vi "AlliGator n-Exp + IRF Fit v4.vi"(0 "Decay":cluster{"t Array":dbl[], "Data Array":dbl[]}, 1 "VI Refnum":refnum<vi>, 5 "IRF":cluster{"t Array":dbl[], "IRF Array":dbl[]}, 7 "Fit Options":T13={"Show Fit Residuals"=TRUE, "Fit Model"=enum."1-Exponential", "Residual Type"=enum."Standard", "Max Decay Percentile"=0.0, "Min Decay Percentile"=0.0, "Show Full Decay"=TRUE, "Weights"=enum."Unweighted", "Fitting Method"=enum."Least Square", "Compute Parameter Uncertainties"=TRUE, "Periodic Boundaries"=TRUE, "Model Calculation"=enum."Simulation", "Period"=1.2500000000000001e-08, "Termination Criteria"={"Max Iterations"=1000, "Max Function Calls"=0, "Max Time"=1000.0, "Function Tolerance"=1e-06, "Parameter Tolerance"=1e-06, "Gradient Tolerance"=0.0, "Min Lambda"=1e-06, "Max Lambda"=1e-06, "Initial Tick Count"=0}, "Offset Resolution"=1.2500000000000001e-08, "Use Local IRF"=TRUE, "Fitting Algorithm"=enum."Levenberg-Marquardt"} {"Offset Resolution" min=0.0; "Period" min=0.0; "Min Decay Percentile" min=0.0 max=1.0; "Max Decay Percentile" min=0.0 max=1.0}, 9 "MLE Fit Options":T1, 11 "error in (no error)":errorcluster, 12 "All Parameter Constraints":T10) -> (3 "All unscaled Fit Parameters (w tau)":dbl[](array[numeric]), 4 "Fitted Decay":cluster{"t Array":dbl[], "Fitted Array":dbl[]}, 6 "Residuals":cluster{"t Array":dbl[], "Residual Array":dbl[]}, 8 "Fit Output":T4={"best nonlinear fit"=[], "best fit parameters"=[], "R^2"=0.0, "RMSE"=0.0, "error out"={"status"=FALSE, "code"=0, "source"=""}, "Fitting Method"=enum."Least Square", "number of function calls"=0, "number of iterations"=0, "covariance"=[], "Chi 2"=0.0, "DOF"=0, "Fit Convergence Criterion"=enum."Continue", "Fitting Algorithm"=enum."Levenberg-Marquardt", "Weighted Fit"=FALSE, "Gradient"=0.0, "|Delta Chi 2|"=0.0, "|Delta Chi 2|/Chi 2"=0.0, "Max |Delta a| /|a|"=0.0, "Lambda"=-1.0, "RSS"=0.0, "AIC"=0.0, "BIC"=0.0, "Max number of function calls"=0, "Max number of iterations"=0, "IRF"={"X Array"=[], "Y Array"=[]}, "IRF Normalization Factor"=0.0, "Decay Normalization Factor"=0.0}, 10 "Delta Best Fit Parameters (w tau)":dbl[](array[numeric]), 13 "Guess Parameters Options":T3=enum."User-provided (normalized)", 14 "Guess Parameters":dbl[](array[numeric]), 15 "error out":errorcluster)   [LabVIEW 2021, in "AlliGator Decay Analysis.lvlib" / "AlliGator Decay Fit.lvlib"]
doc: "Fits the provided decay to 1-Exp or 2-Exp model.\n\nThis VI assumes that <B>All Parameter Constraints</B> involve tau (rather than the square root of lifetime) and returns values with the same assumption."
uses:
  AlliGator Decay Fit.lvlib
  Fits/IRF(X)PSED/Decay Fit Options v2.ctl
  Fits/Decay Convolution/Decay Model.ctl
  Fits/Residual Type.ctl
  Fits/IRF(X)PSED/Fit Weights Type.ctl
  Fits/Non-linear Fitting Method v2.ctl
  Fits/Fit Calculation Method.ctl
  Fits/Non-linear Fitting Algorithm.ctl
  Fits/IRF(X)PSED/Decay Fit Parameter Constraints Arrays.ctl
  Fits/IRF(X)PSED/Decay Fit Parameters In List.ctl
  Fits/Non-linear Fit Output v3.ctl
  Fits/Nonlinear Fit Method.ctl
  <vilib>/Analysis/Matrix/Datatypes/RealMatrix.ctl
  Fits/Convergence Criteria.ctl
  Graphs/XY Graph/XY Plot Data.ctl
  AlliGator Guess Parameters Options.ctl
  Fits/IRF(X)PSED/MLE Fit Options.ctl
  Fits/IRF(X)PSED/MLE Baseline Offset Type.ctl
  Fits/Decay Convolution/Fit Control Data v2.ctl
  Fits/Decay Fit Steps.ctl
  Fits/Fit Results (statistics).ctl
  AlliGator Variables List.ctl
  Fits/Abort Fit Global.vi
  <vilib>/Utility/error.llb/Error Cluster From Error Code.vi
  <vilib>/ErrorRing/Error Ring.xnode
  Time/Time.lvlib
  Fits/Fits.lvlib
  AlliGator Settings.lvlib
  AlliGator Settings List.ctl
  AlliGator Globals, Variables & Constants.lvlib
  Graphs/XY Graph/XY Graph Add-Ons.lvlib
  <vilib>/Analysis/Matrix/NI_Matrix.lvlib
  Utilities/Utilities.lvlib
  Error/Error.lvlib
panel:
  out "CPU (s)":dbl
  out "XY Graph":T18(graph)
  # "Offset\nBaseline\nAmplitude\nLifetime"
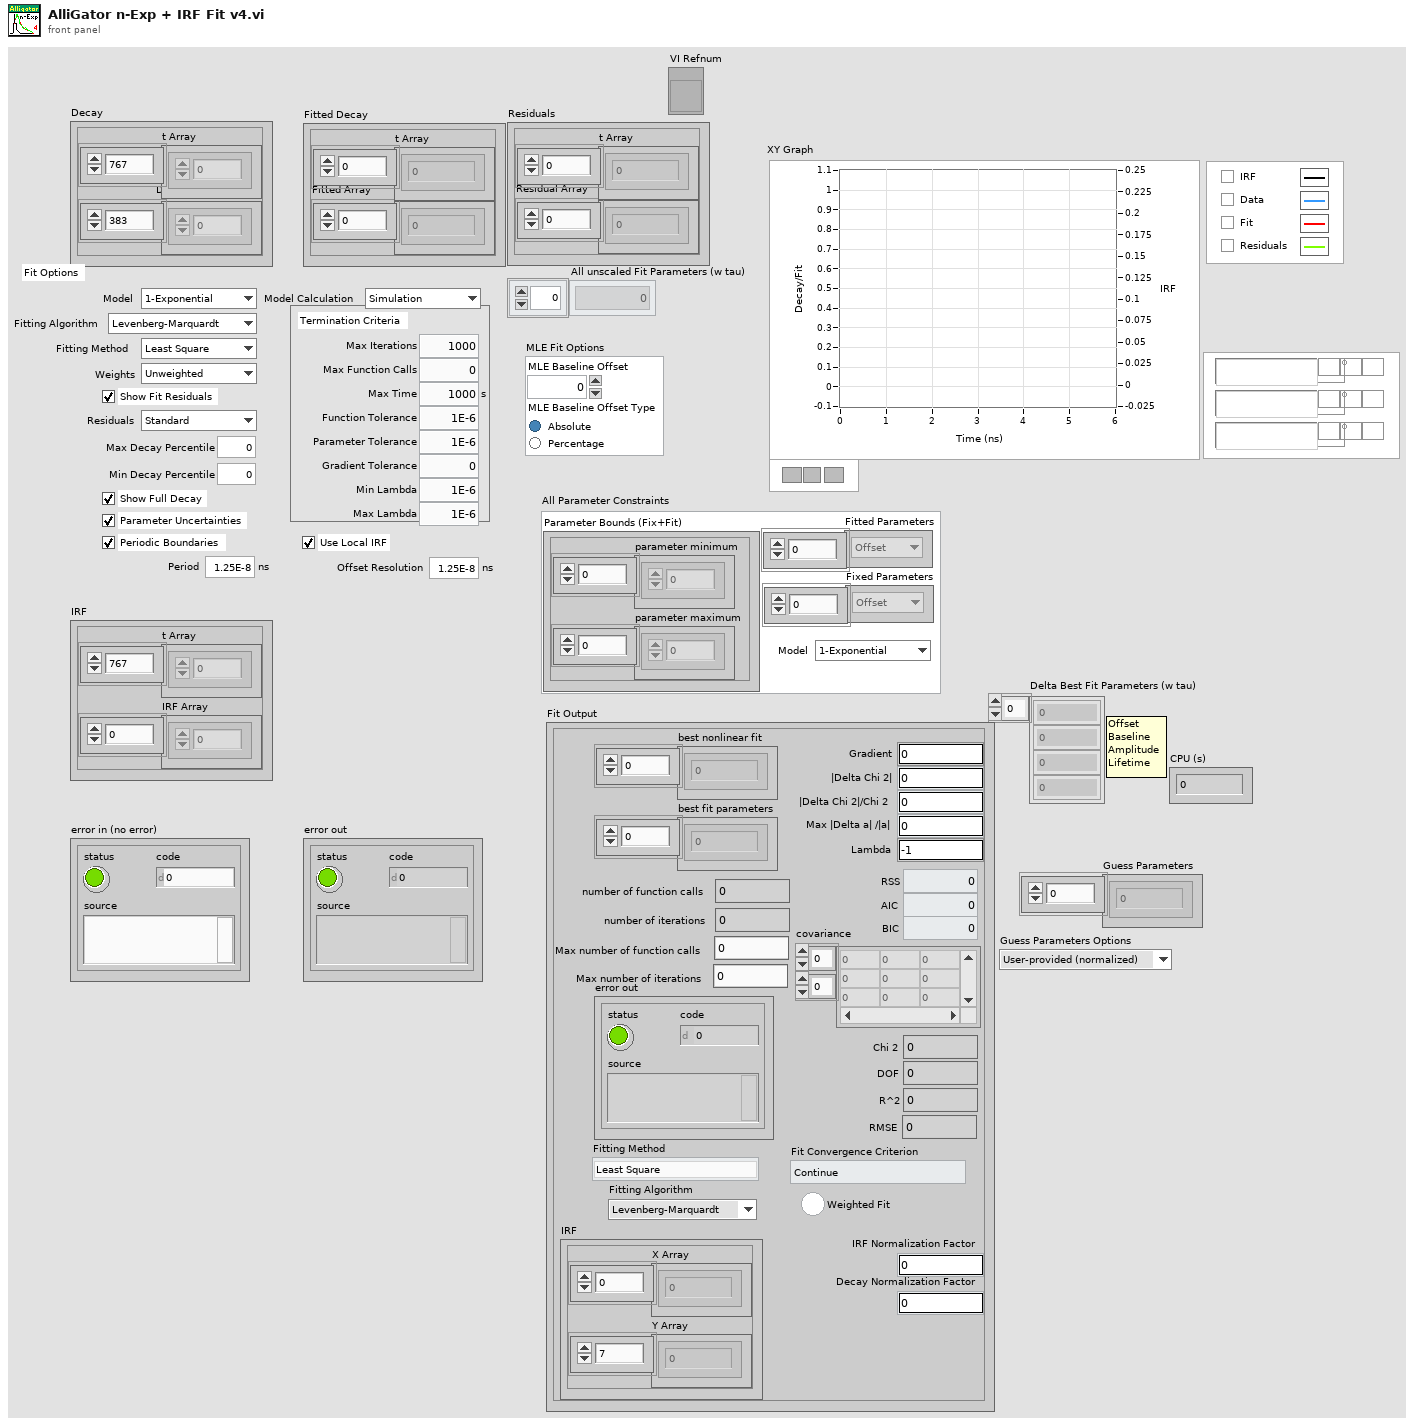
[diagram p1: front panel]
types:
  T1 = typedef "Fits.lvlib/MLE Fit Options.ctl" = cluster{"MLE Baseline Offset":dbl, "MLE Baseline Offset Type":T2}
  T2 = typedef "Fits.lvlib/MLE Baseline Offset Type.ctl" = enum32{"Absolute", "Percentage"}
  T3 = typedef "AlliGator Decay Analysis.lvlib/AlliGator Decay Fit.lvlib/AlliGator Guess Parameters Options.ctl" = enum16{"Numerically estimated", "User-provided", "User-provided (normalized)", "Last valid fitted parameters"}
  T4 = typedef "Fits.lvlib/Non-linear Fit Output v3.ctl" = cluster{"best nonlinear fit":dbl[], "best fit parameters":dbl[], "R^2":dbl, "RMSE":dbl, "error out":errorcluster, "Fitting Method":T5, "number of function calls":i32, "number of iterations":i32, "covariance":T6, "Chi 2":dbl, "DOF":i32, "Fit Convergence Criterion":T7, "Fitting Algorithm":T8, "Weighted Fit":bool, "Gradient":dbl, "|Delta Chi 2|":dbl, "|Delta Chi 2|/Chi 2":dbl, "Max |Delta a| /|a|":dbl, "Lambda":dbl, "RSS":dbl, "AIC":dbl, "BIC":dbl, "Max number of function calls":i32, "Max number of iterations":i32, "IRF":T9, "IRF Normalization Factor":dbl, "Decay Normalization Factor":dbl}
  T5 = typedef "Fits.lvlib/Nonlinear Fit Method.ctl" = enum16{"Least Square", "Least Absolute Residual", "Bisquare", "MLE"}
  T6 = typedef "NI_Matrix.lvlib/RealMatrix.ctl" = dbl[][]
  T7 = typedef "Fits.lvlib/Convergence Criteria.ctl" = enum16{"Continue", "Tolerances Exceeded", "Max Time Exceeded", "Max Iterations Exceeded", "Max Function Evaluations Exceeded", "Scale Range Exceeded"}
  T8 = typedef "Fits.lvlib/Non-linear Fitting Algorithm.ctl" = enum16{"Levenberg-Marquardt", "Trust-Region Dogleg"}
  T9 = typedef "XY Graph Add-Ons.lvlib/XY Plot Data.ctl" = cluster{"X Array":dbl[], "Y Array":dbl[]}
  T10 = typedef "Fits.lvlib/Decay Fit Parameter Constraints Arrays.ctl" = cluster{"Parameter Bounds (Fix+Fit)":cluster{"parameter minimum":dbl[], "parameter maximum":dbl[]}, "Fitted Parameters":T11[], "Fixed Parameters":T11[], "Fit Model":T12}
  T11 = typedef "Fits.lvlib/Decay Fit Parameters In List.ctl" = enum16{"Offset", "Baseline", "A_1", "tau_1", "A_2", "tau_2"}
  T12 = typedef "Fits.lvlib/Decay Model.ctl" = enum16{"1-Exponential", "2-Exponentials"}
  T13 = typedef "Fits.lvlib/Decay Fit Options v2.ctl" = cluster{"Show Fit Residuals":bool, "Fit Model":T12, "Residual Type":T14, "Max Decay Percentile":dbl, "Min Decay Percentile":dbl, "Show Full Decay":bool, "Weights":T15, "Fitting Method":T16, "Compute Parameter Uncertainties":bool, "Periodic Boundaries":bool, "Model Calculation":T17, "Period":dbl[unit], "Termination Criteria":cluster{"Max Iterations":i32, "Max Function Calls":i32, "Max Time":dbl[unit], "Function Tolerance":dbl, "Parameter Tolerance":dbl, "Gradient Tolerance":dbl, "Min Lambda":dbl, "Max Lambda":dbl, "Initial Tick Count":u32}, "Offset Resolution":dbl[unit], "Use Local IRF":bool, "Fitting Algorithm":T8}
  T14 = typedef "Fits.lvlib/Residual Type.ctl" = enum16{"Standard", "Normalized", "Reduced"}
  T15 = typedef "Fits.lvlib/Fit Weights Type.ctl" = enum16{"Unweighted", "1/Variance", "Best of All"}
  T16 = typedef "Fits.lvlib/Non-linear Fitting Method v2.ctl" = enum16{"Least Square", "Least Absolute Residual", "Bisquare", "MLE", "-", "Best of All"}
  T17 = typedef "Fits.lvlib/Fit Calculation Method.ctl" = enum16{"Simulation", "Convolution", "Integration"}
  T18 = cluster{"t Array":dbl[], "best nonlinear fit":dbl[]}[]
  T19 = typedef "Fits.lvlib/Fit Control Data v2.ctl" = cluster{"IRF":T9, "Laser Period":dbl, "SYNC Period":dbl, "Fixed Parameter Names":T11[], "Fixed Parameter Values":dbl[], "Fitted Parameter Names":T11[], "Fit Model":T12}
  T20 = cluster{"Max Iterations":i32, "Max Function Calls":i32, "Max Time":dbl[unit], "Function Tolerance":dbl, "Parameter Tolerance":dbl, "Gradient Tolerance":dbl, "Min Lambda":dbl, "Max Lambda":dbl, "Initial Tick Count":u32}
  T21 = cluster{"parameter minimum":dbl[], "parameter maximum":dbl[]}
  T22 = typedef "AlliGator Settings.lvlib/AlliGator Settings List.ctl" = enum16{"GUI:Visible Settings Tab", "GUI:Last Run Version", "Source Image:Use Image Histogram for Contrast", "Source Image:Low Count Pixels Rejection Options", "Source Image:High Count Pixels Rejection Options", "Source Image:Use Image Brightness", "Source Image:Blend Overlay with Image Background", "Source Image:Use Fixed ROI Diameter", "Source Image:ROI Diameter", "Source Image:ROI Center Color", "Source Image:Peak Threshold", "Source Image:Intensity Threshold", "Source Image:Image Binning Options", "Source Image:Image Smoothing Options", "Source Image:Image Histogram Active", "Source Image:Invert Binary Mask", "Source Image:Hot Pixel Removal", "Source Image:Overlay Analyzed ROI Center", "Source Image:Auto-Adjust Contrast", "Source Image:Histogram Lower Percentile", "Source Image:Histogram Upper Percentile", "Source Image:Save Source Image", "Source Image:Scale Bar Options", "Source Image:Image Resolution (Pixel Size)", "Source Image:Flatfield Correction", "Source Image:Show Dead Left Columns Correction", "Source Image:Dead Left Columns Correction", "Source Image:Image Pre-Processing Operations Order", "Data Information:Gate Width", "Data Information:Nanotime Gate Separation", "Data Information:Macrotime Gate Separation", "Data Information:Gate Step", "Data Information:# Gates", "Data Information:Gate Image Exposure", "Data Information:Gate Image Integration", "Data Information:Gates to Skip", "Data Information:Gates to Keep", "Data Information:Define Gates to", "Data Information:Channel Name", "Data Information:Available Channel Names", "Data Information:Channel Arithmetic", "Data Information:Background File Subtraction", "Data Information:Background File", "Data Information:Background Scaling Factor", "Data Information:Background Pile-up Correction", "Data Information:Background Pixel Well Capacity", "Data Information:Laser Period", "Data Information:SYNC Period", "Data Information:Pile-up Correction", "Data Information:Pixel Well Capacity", "Data Information:Dataset Scaling Factor", "Fluorescence Decay_Decay Pre-Processing:Reverse Gates", "Fluorescence Decay_Decay Pre-Processing:Verbose Decay Pre-Processing", "Fluorescence Decay_Decay Pre-Processing:Use Decay Pre-Processing", "Fluorescence Decay_Decay Pre-Processing:Background Subtraction", "Fluorescence Decay_Decay Pre-Processing:Background Definition Range", "Fluorescence Decay_Decay Pre-Processing:Baseline Subtraction Method", "Fluorescence Decay_Decay Pre-Processing:Decay Pre-Processing Operations Order", "Fluorescence Decay_Decay Pre-Processing:Smoothing Parameter", "Fluorescence Decay_Decay Pre-Processing:Shift Decay", "Fluorescence Decay_Decay Pre-Processing:Decay Shift Parameters", "Fluorescence Decay_Decay Pre-Processing:Fold Decay", "Fluorescence Decay_Decay Pre-Processing:# Folds", "Fluorescence Decay_Decay Pre-Processing:1-Normalize Decay", "Fluorescence Decay_Decay Pre-Processing:[0-1]-Normalize Decay", "Fluorescence Decay_Decay Pre-Processing:Smoothen Decay", "Fluorescence Decay_Decay Pre-Processing:Extrapolate Decay", "Fluorescence Decay_Decay Pre-Processing:Use Periodicity", "Fluorescence Decay_Decay Pre-Processing:Use Cursors", "Fluorescence Decay_Decay Pre-Processing:Tail Fraction", "Fluorescence Decay_Decay Pre-Processing:Head Fraction", "Fluorescence Decay_Decay Pre-Processing:Additional Points", "Fluorescence Decay_Decay Pre-Processing:Straighten Decay", "Fluorescence Decay_Decay Pre-Processing:Constant Background", "Fluorescence Decay_Decay Pre-Processing:Pixel-Normalize Decay", "Fluorescence Decay_Advanced Analysis:Extract IRF instead of Decay", "Fluorescence Decay_Advanced Analysis:IRF Extraction Options", "Fluorescence Decay_Advanced Analysis:IRF Optimization Options", "Fluorescence Decay_Advanced Analysis:Square Pulse Options", "Fluorescence Decay_Advanced Analysis:IRF Order", "Fluorescence Decay_Advanced Analysis:IRF Time Constants", "Fluorescence Decay_Advanced Analysis:Wavelet Analysis Options", "Fluorescence Decay_Advanced Analysis:Average Lifetime Options", "Fluorescence Decay_Fit Options:Fit Options", "Fluorescence Decay_Fit Options:Use Legacy Fitting Approach", "Fluorescence Decay_Fit Options:Use Data Information Laser Period", "Fluorescence Decay_Fit Parameters:Displayed Fit Parameters", "Fluorescence Decay_Fit Parameters:Fit Parameter Constraints", "Fluorescence Decay_Fit Parameters:Export Tabulated Results", "Fluorescence Decay_Fit Parameters:MLE Baseline Offset Type", "Fluorescence Decay_Fit Parameters:MLE Baseline Offset", "Fluorescence Decay_Fit Parameters:Guess Parameter Names", "Fluorescence Decay_Fit Parameters:Guess Parameter Values", "Fluorescence Decay_Fit Parameters:Guess Parameters Options", "Fluorescence Decay_Styles:Show Last Decay Only", "Fluorescence Decay_Styles:Decay Graph Color Array", "Fluorescence Decay:Decay Graph Active", "Fluorescence Decay Statistics:Min Peak Value", "Fluorescence Decay Statistics:Reject Low Decay Peak Pixels", "Fluorescence Decay Statistics:Reject High Decay Peak Pixels", "Fluorescence Decay Statistics:Max Peak Value", "Time Traces:Use File Timestamp", "Time Traces:Time Step", "Time Traces:Use Intensity Correction File", "Time Traces:Intensity Correction File", "Phasor Plot:Phasor Plot Smoothing Options", "Phasor Plot:Phasor Plot Size", "Phasor Plot:Phasor Plot Graphics Options", "Phasor Plot:Cumulative Phasor Plot", "Phasor Plot:Use Phasor Brightness", "Phasor Plot:Blend Overlay with Phasor Background", "Phasor Plot:Save Phasor Plot", "Phasor Plot:Show References", "Phasor Plot:Phasor Ratio Decay Range", "Phasor Plot:Exponential Fading", "Phasor Plot:Phasor Ratio Reference Colors", "Phasor Plot:Reference Radius", "Phasor Plot:Show Color Map Vertices", "Phasor Plot:Phasor Plot Active", "Phasor Plot:Phasor Ratio Color Map Type", "Phasor Plot:Phasor Ratio Color Map", "Phasor Plot:Phasor Ratio Display Range", "Phasor Plot:Selected Image ROI(s)", "Phasor Plot:All Image ROIs", "Phasor Plot:Selected Phasor Plot ROI(s)", "Phasor Plot:All Phasor Plot ROIs", "Phasor Plot:Phasor Ratio Color-Coded Quantity", "Phasor Plot:Store Phasor Harmonics", "Phasor Plot:Draw Reference Segment", "Phasor Plot:User-Defined Quantity", "Phasor Graph:Phasor Frequency", "Phasor Graph:Phasor Ratio Type", "Phasor Graph:Pixel-level Phasor Computation", "Phasor Graph:Save Phasor Graph", "Phasor Graph:Phasor Graph Active", "Phasor Graph:Phasor SDV Options", "Phasor Calibration:Use Backup Calibration if needed", "Phasor Graph:Define Shortest Lifetime as", "Phasor Calibration:Backup Calibration Type", "Phasor Calibration:Calibration Type", "Phasor Calibration:Calibration Lifetime", "Phasor Calibration:Calibration Map Algorithm", "Single-Exponential Phasor Locus (SEPL):Gate Parameters", "Single-Exponential Phasor Locus (SEPL):User-defined Gate", "Single-Exponential Phasor Locus (SEPL):User-defined IRF", "Single-Exponential Phasor Locus (SEPL):Phasor Parameters", "Single-Exponential Phasor Locus (SEPL):Decay & IRF Parameters", "Single-Exponential Phasor Locus (SEPL):Display Parameters", "Lifetime Analysis:Decay Analysis Parameters", "Lifetime Analysis:Lifetime Map Active", "Plugins:Python Settings", "Miscellaneous:Verbose Mode", "Miscellaneous:Beep after Script", "Miscellaneous:Saved Image File Format", "Miscellaneous:Exported Gate Image Settings", "Miscellaneous:Include Loading in Timing", "Miscellaneous:Verbose Settings Mode", "Miscellaneous:Histogram Options", "Miscellaneous:Beep on Error", "Miscellaneous:# Logical Processors Used", "Miscellaneous:ROI Description Max Characters", "Miscellaneous:Verbose Error Mode", "Miscellaneous:Transparent Mask Color"}
  T23 = typedef "Fits.lvlib/Decay Fit Steps.ctl" = enum16{"Unweighted Fit", "Weighted Fit", "Best Fit"}
  T24 = typedef "Fits.lvlib/Decay Fit Parameter Constraints with Values.ctl" = cluster{"Fitted parameter bounds":cluster{"parameter minimum":dbl[], "parameter maximum":dbl[]}, "Fixed Parameter Values":dbl[], "Fixed Parameter Names":T11[], "Fitted Parameter Names":T11[], "Fit Model":T12}
  T25 = typedef "Fits.lvlib/Fit Results (statistics).ctl" = cluster{"Chi2/DOF":dbl, "R2":dbl, "RMSE":dbl, "Fitting Method":T16, "Fitting Algorithm":T8}
  T26 = typedef "AlliGator Globals, Variables & Constants.lvlib/AlliGator Variables List.ctl" = enum16{"---- GUI ----", "Initialization Status", "State Indicators Refnum", "Original AlliGator Menu Items", "Current Action Loop State", "Script in progress", "Playback", "Loop Playback", "Search ROI Used", "Search ROI", "Decay Graph Max Legend Size", "Intensity Graph Max Legend Size", "Decay Statistics Graph Max Legend Size", "Phasor Graph Max Legend Size", "Phasor Ratio Graph Max Legend Size", "Lifetime Graph Max Legend Size", "---- Files ----", "Export Dataset Frames as Individual Files", "Show Batch Export Help Balloons", "Frames in Dataset", "ptu File Frame Start Indices", "Current Frame in Dataset", "Current Frame Timestamp", "------ Python Plugins ------", "Python Plugins Information", "Python Session", "Valid Python Session?", "---- Source Image ----", "Dataset Loaded", "Dataset Metadata", "Dataset Channel", "Dataset Data Description", "Background Dataset Metadata", "Background Dataset Channel", "Background Dataset Data Description", "Background File Subtraction", "Background File Path", "Background File Pile-up Correction", "Background File Pixel Well Capacity", "Background File Scaling Factor", "Source Image ROIs", "Current Source Image ROI", "Source Image ROI Event Refnum", "X_Source Image Display Range", "X_Source Image Palette Information", "Source Image Palette List", "Source Image Scale", "Current Dataset Load Settings", "Source Image:ROI Overlay Color", "---- Image Profile Window ----", "Image Profile:Overlay ROI in Source Image", "Image Profile Window Event Refnum", "Image Profile:IntensityType", "Image Profile:Intensity Average Type", "Image Profile:Intensity-weighted SDV", "Image Profile:Box Profile Type", "Image Profile Window Open", "Image Profile:Plotted Fit Parameter", "X_Type of Displayed Image", "X_Time Gate Slider", "Dataset Path", "Source Image Overlay to Erase", "Is Displayed Image Accumulated", "White Light Image Modified", "Mask Image Modified", "Macrotime Gate Separation", "------ Phasor Graph -------", "Phasor Graph:Show Line", "---- Phasor Plot ---", "Phasor Plot Parameters Changed", "FLI Dataset Modified since last Phasor Plot Calculation", "Phasor Harmonics Data", "Selected Phasor Harmonics", "Phasor Harmonic Manager Event Refnum", "Phasor Plot ROIs", "Current Phasor Plot ROI", "Phasor Plot ROI Event Refnum", "Phasor Plot Image Reference Points", "Phasor Plot Computed", "Phasor Plot Palette Information", "Phasor Plot Palette List", "Phasor Ratio Palette Information", "Phasor Ratio Palette List", "Phasor Image Scale", "Phasor Plot Image Overlay to Erase", "Phasor Plot Image Elements to Update", "Current Phasor Plot Calculation Parameters", "Current Phasor Calibration Options", "Reset Cumulated Phasor Plot", "Phasor Ratio Reference 1", "Phasor Ratio Lifetime Reference 1", "Phasor Ratio Reference 1 Frequency", "Phasor Ratio Reference 2", "Phasor Ratio Lifetime Reference 2", "Phasor Ratio Reference 2 Frequency", "---- Decay Analysis ----", "Number of Selected Decays to Fit", "LS Fit Results", "LAR Fit Results", "BS Fit Results", "Last Decay Max - Min", "Best Fit Parameters", "Best Fit Parameter Names", "Actual Size X", "Actual Size Y", "Binning X", "Binning Y", "Actual # Gates", "Dataset Number", "Gates to...", "Gates Skipped", "Gates to keep", "Gate Step", "Gate Separation", "Reversed Gates", "Pile-up Correction", "Pixel Well Capacity", "Background Subtracted", "Background Subtraction Method", "Background Definition Range", "Background File (deprecated)", "Number of Dataset Accumulated", "Array of Accumulated Dataset Paths", "Do Averaged Datasets", "Destination File Path", "Process Plot Target", "Use 1/D as Phasor Frequency", "---- Decay Fit Parameter Map -----", "Decay Fit Parameter Map Palette Information", "Decay Fit Parameter Map Palette List", "Local Decay Graph Window Event Refnum", "------- Local Decay Window ---------", "Use normalized IRF for convolution", "----- Miscellaneous ----", "Skippable Dialog Windows Status"}
  T27 = cluster{"t Array":dbl[], "best nonlinear fit":dbl[]}
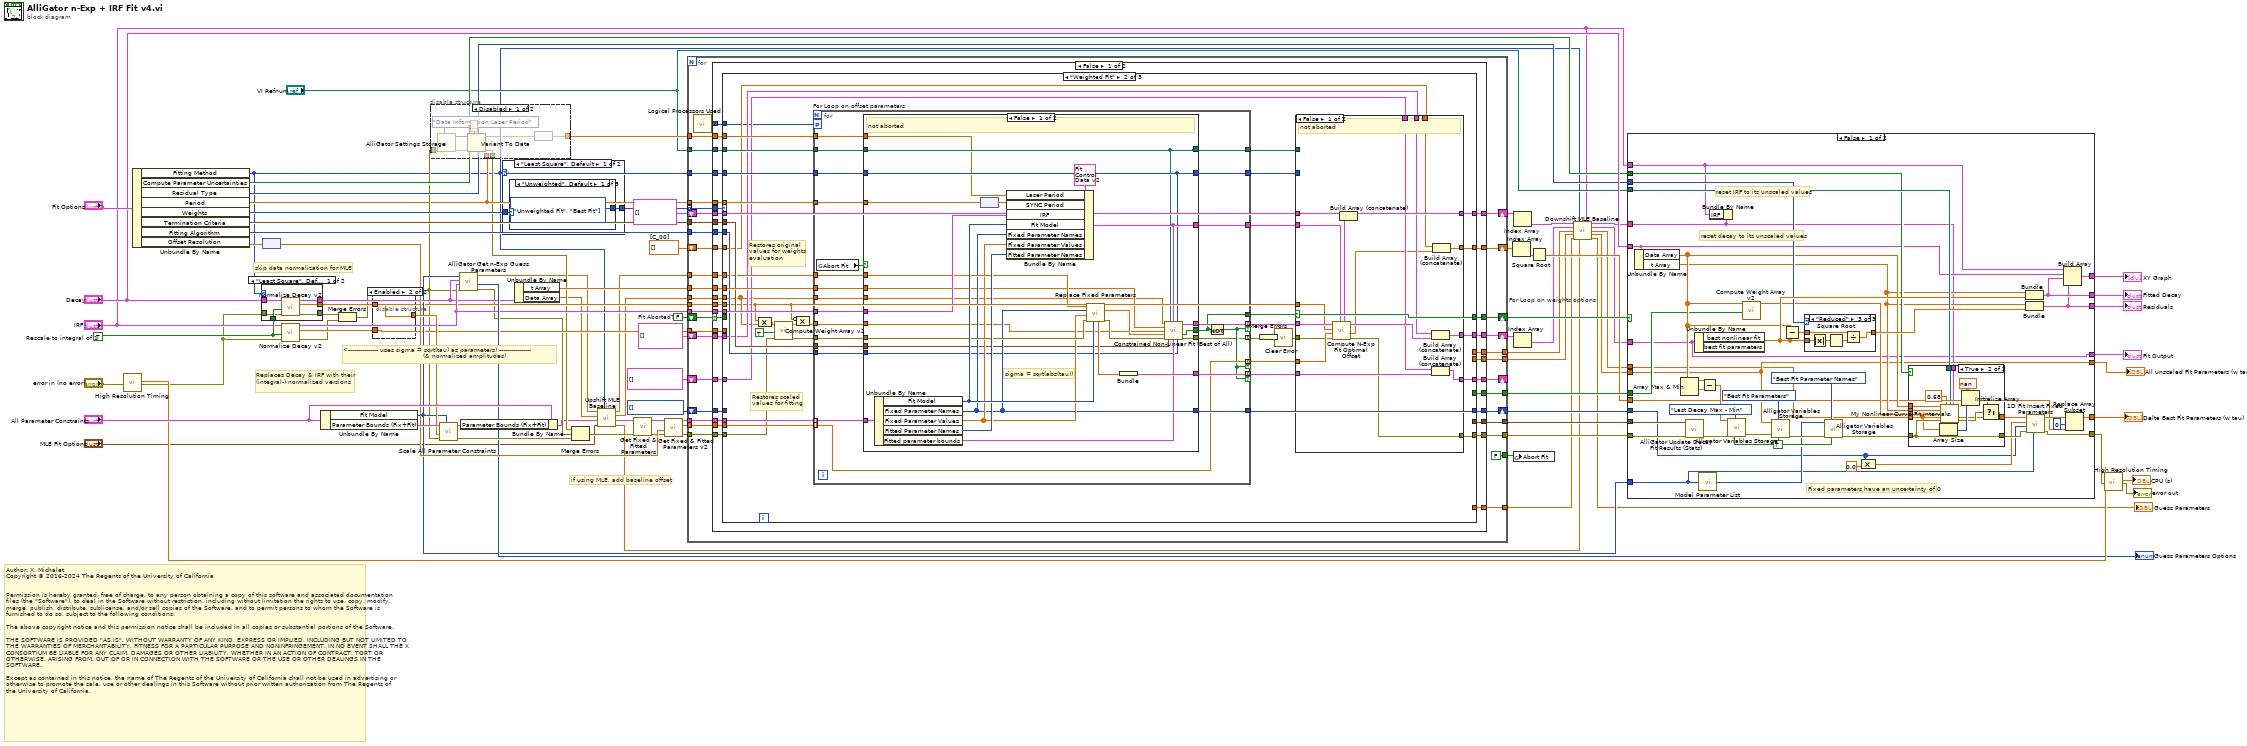
[diagram p0: block diagram]
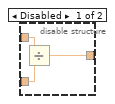
[diagram p2: hidden frame]
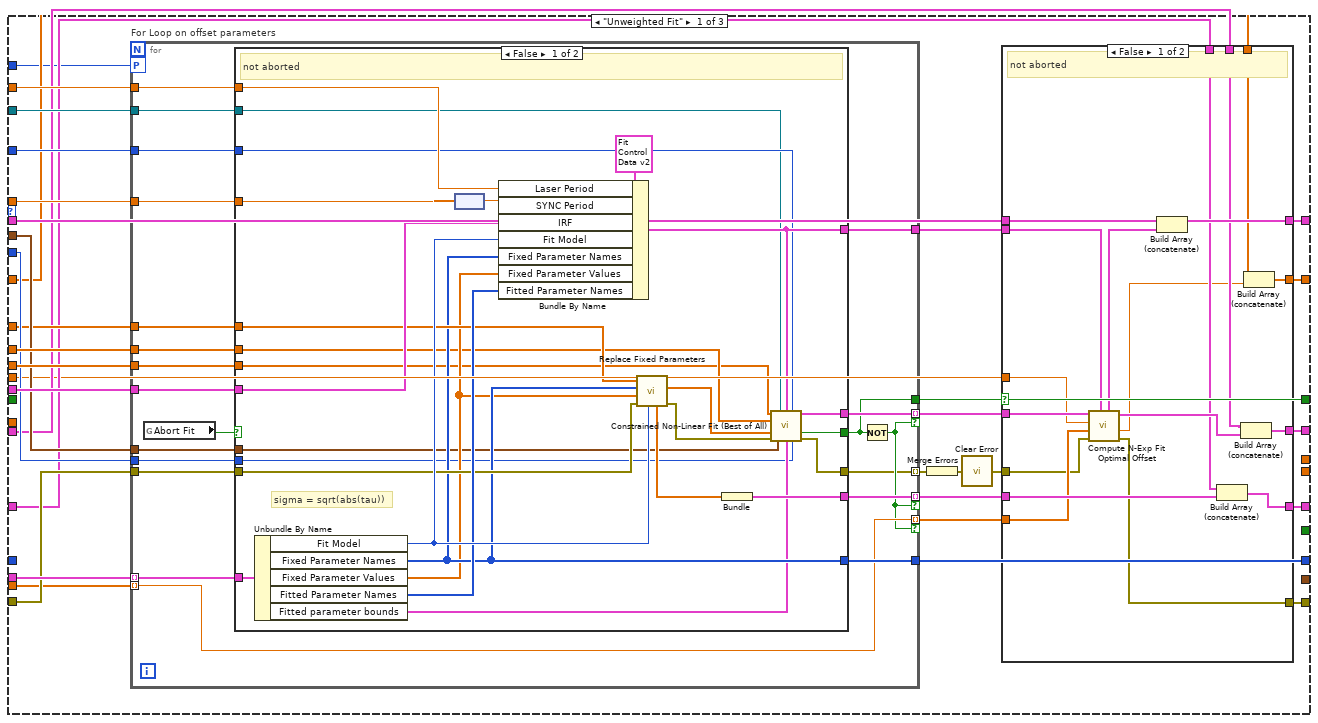
[diagram p3: hidden frame]
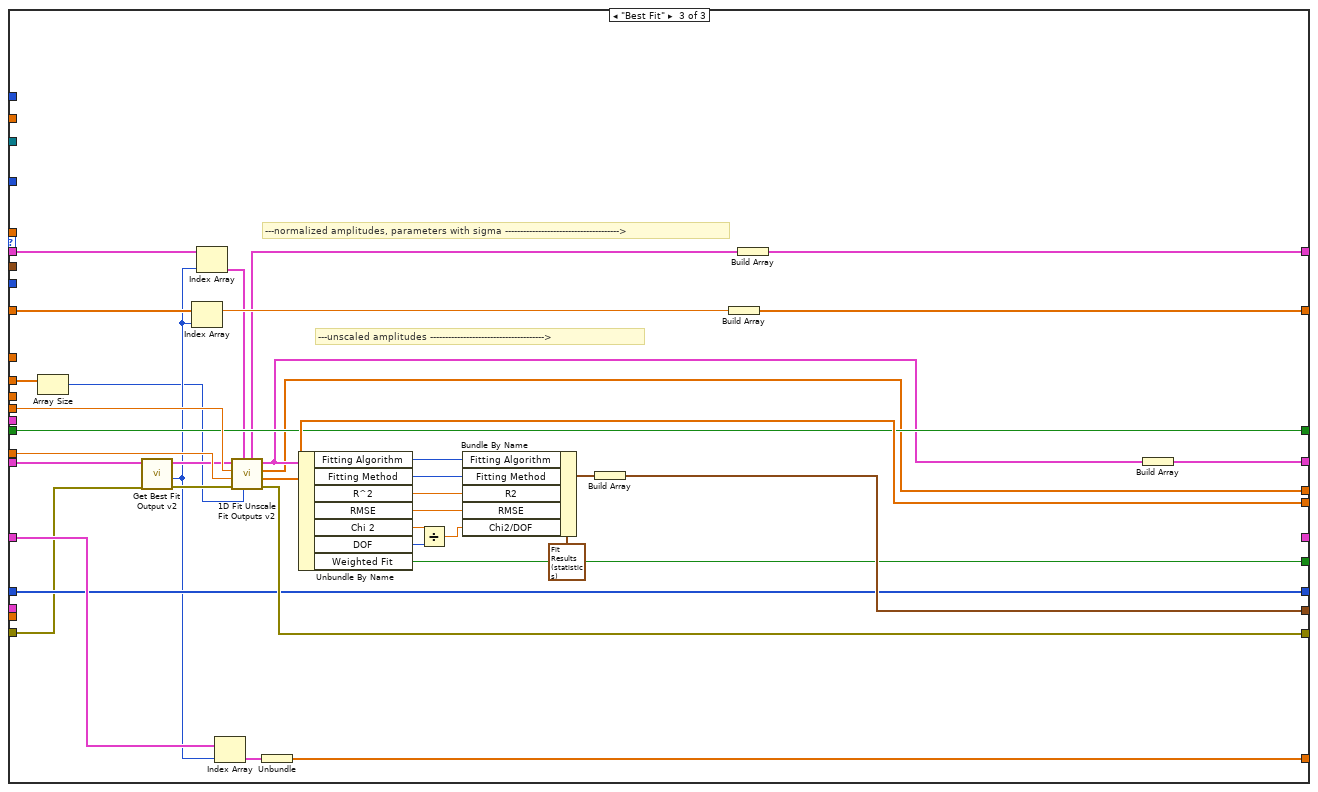
[diagram p8: hidden frame]
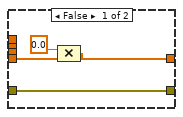
[diagram p10: hidden frame]
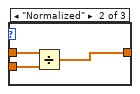
[diagram p12: hidden frame]
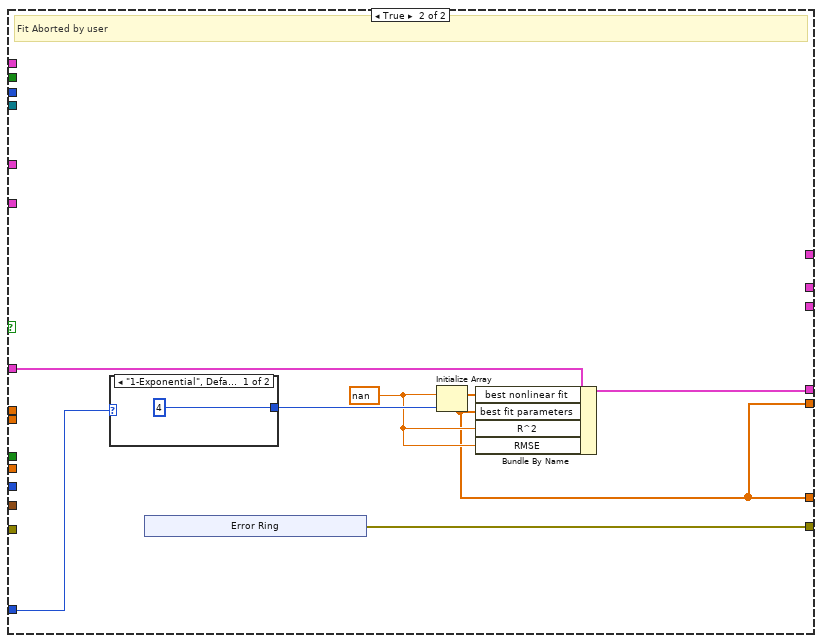
[diagram p13: hidden frame]
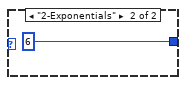
[diagram p14: hidden frame]
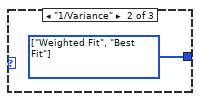
[diagram p15: hidden frame]
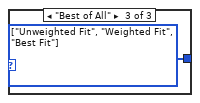
[diagram p16: hidden frame]
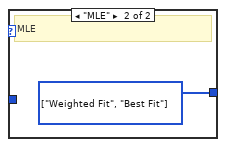
[diagram p17: hidden frame]
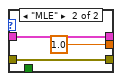
[diagram p18: hidden frame]
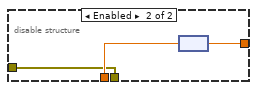
[diagram p19: hidden frame]
diagram:
  w40 = dbl[] []  # [C_00]
  w42 = T11[] [] items=["Offset", "Baseline", "A_1", "tau_1", "A_2", "tau_2"] ("Fixed Parameter Names")
  w56 = FALSE  # Fit Aborted?
  w30 = TRUE  # Rescale to integral of 1
  # "Author: X. Michalet\nCopyright © 2016-2024 The Regents of the University of California\n \n\nPermission is hereby granted, free of charge, to any person obtaining a copy of this software and associated documentation files (the \"Software\"), to deal in the Software without restriction, including without limitation the rights to use, copy, modify, merge, publish, distribute, sublicense, and/or sell copies of the Software, and to permit persons to whom the Software is furnished to do so, subject to the following conditions:\n\nThe above copyright notice and this permission notice shall be included in all copies or substantial portions of the Software.\n\nTHE SOFTWARE IS PROVIDED \"AS IS\", WITHOUT WARRANTY OF ANY KIND, EXPRESS OR IMPLIED, INCLUDING BUT NOT LIMITED TO THE WARRANTIES OF MERCHANTABILITY, FITNESS FOR A PARTICULAR PURPOSE AND NONINFRINGEMENT. IN NO EVENT SHALL THE X CONSORTIUM BE LIABLE FOR ANY CLAIM, DAMAGES OR OTHER LIABILITY, WHETHER IN AN ACTION OF CONTRACT, TORT OR OTHERWISE, ARISING FROM, OUT OF OR IN CONNECTION WITH THE SOFTWARE OR THE USE OR OTHER DEALINGS IN THE SOFTWARE.\n\nExcept as contained in this notice, the name of The Regents of the University of California shall not be used in advertising or otherwise to promote the sale, use or other dealings in this Software without prior written authorization from The Regents of the University of California."
  # "if using MLE, add baseline offset"
  # "skip data normalization for MLE"
  # "Replaces Decay & IRF with their (integral-) normalized versions"
  # "<--------------- uses sigma = sqrt(tau) as parameters) ----------------\n                                        (& normalized amplitudes)"
  n1 = call "High Resolution Timing.vi"("Error In"="error in (no error)") -> ("elapsed (relative) seconds"=w63:dbl, "Error Out"=w4:errorcluster)  [unwired: 16 in, 1 out]
  n2 = Unbundle By Name("Fit Options") -> ("Fitting Method"=w7:T16, "Compute Parameter Uncertainties"=w59:bool, "Residual Type"=w58:T14, "Period"=w28:dbl[unit], "Weights"=w65:T15, "Termination Criteria"=w62:T20, "Fitting Algorithm"=w61:T8, "Offset Resolution"=w54:dbl[unit])
  n3 = case shown="\"Least Square\", Default" w7 {
    tunnel: "Decay" -> [w92 w95]
    tunnel: [w91 w95] -> w46
    tunnel: [w90 1.0 ("Normalization Factor")] -> w32
    tunnel: w30 -> [w89 _]
    tunnel: w4 -> [w88 w93]
    tunnel: [w87 w93] -> w25
    frame "Least Square", Default {
      n4 = call "Normalize Decay v2.vi"("Error In"=w88, "Max = 1 (F)/Integral = 1 (T)"=w89, "Decay"=w92) -> ("Error Out"=w87:errorcluster, "Normalization Factor"=w90:dbl, "Normalized Decay"=w91:cluster{"t Array":dbl[], "Y Array":dbl[]})  [unwired: 4 in, 2 out]
    }
    frame "MLE" {
    }
  }
  n5 = node(w54) -> (w53:dbl)
  n6 = call "Normalize Decay v2.vi"("Error In"=w4, "Max = 1 (F)/Integral = 1 (T)"=w30, "Decay"="IRF") -> ("Error Out"=w26:errorcluster, "Normalization Factor"=w31:dbl, "Normalized Decay"=w47:cluster{"t Array":dbl[], "Y Array":dbl[]})  [unwired: 4 in, 2 out]
  n7 = Unbundle By Name("All Parameter Constraints") -> ("Fit Model"=w45:T12, "Parameter Bounds (Fix+Fit)"=w75:T21)
  n8 = Merge Errors(w25, w26) -> (w29:errorcluster)
  n9 = disable-structure shown="Enabled" {
    disable-tunnel: [w98 w99] -> w71
    disable-tunnel: w32 -> [w97 w99]
    disable-tunnel: w31 -> [w96 _]
    frame Disabled {
      n10 = Divide(x=w97, y=w96) -> (x/y=w98:dbl)
    }
    frame Enabled {
    }
  }
  n11 = disable-structure shown="Disabled" {
    disable-tunnel: [w102 w109] -> w79
    disable-tunnel: [w101 w108] -> w24
    disable-tunnel: w29 -> [w100 w108]
    disable-tunnel: w28 -> [_ w110]
    frame Disabled {
      n12 = call "AlliGator Settings Storage.vi"("AlliGator Settings List"=AlliGator_Settings_List."Data Information:Laser Period", "Error In"=w100) -> ("Error Out"=w105:errorcluster, "Variant Data out"=w106:variant)  [unwired: 8 in]
      n13 = Variant To Data(error in=w105, type=dbl[unit] 1e-09 ("New"), Variant=w106) -> (data=w103:dbl[unit], error out=w101:errorcluster)
      n14 = node(w103) -> (w102:dbl)
    }
    frame Enabled {
      n15 = node(w110) -> (w109:dbl)
    }
  }
  n16 = call "Scale All Parameter Constraints.vi"("Fit Model"=w45, "Error In"=w29, "Normalization Factor"=w71, "parameter bounds in (w tau)"=w75) -> ("Error Out"=w68:errorcluster, "parameter bounds out (w sigma)"=w73:T21)  [unwired: 6 in]
  n17 = call "AlliGator Get n-Exp Guess Parameters.vi"("Error In"=w29, "IRF"=w47, "Decay"=w46, "Fit Model"=w45) -> ("Error Out"=w23:errorcluster, "Guess Parameters Options"=→"Guess Parameters Options":T3, "Guess Parameters"=w13:dbl[])  [unwired: 5 in]
  n18 = Bundle By Name(cluster="All Parameter Constraints", "Parameter Bounds (Fix+Fit)"=w73) -> (w11:T10)
  n19 = case shown="\"Least Square\", Default" w7 {
    tunnel: w65 -> [w112 _]
    tunnel: [w111 w116] -> w64
    frame "Least Square", Default {
      n20 = case shown="\"Unweighted\", Default" w112 {
        tunnel: [w113 w114 w115] -> w111
        frame "Unweighted", Default {
          w113 = T23[] [enum."Unweighted Fit", enum."Best Fit"] items=["Unweighted Fit", "Weighted Fit", "Best Fit"]
        }
        frame "1/Variance" {
          w114 = T23[] [enum."Weighted Fit", enum."Best Fit"] items=["Unweighted Fit", "Weighted Fit", "Best Fit"]
        }
        frame "Best of All" {
          w115 = T23[] [enum."Unweighted Fit", enum."Weighted Fit", enum."Best Fit"] items=["Unweighted Fit", "Weighted Fit", "Best Fit"]
        }
      }
    }
    frame "MLE" {
      w116 = T23[] [enum."Weighted Fit", enum."Best Fit"] items=["Unweighted Fit", "Weighted Fit", "Best Fit"]
      # "MLE"
    }
  }
  n21 = Unbundle By Name(w46) -> ("t Array"=w78:dbl[], "Data Array"=w12:dbl[])
  n22 = Merge Errors(w24, w23, w68) -> (w14:errorcluster)
  n23 = call "Upshift MLE Baseline.vi"("NL Fit Method"=w7, "MLE Fit Options"="MLE Fit Options", "All Parameter Constraints in"=w11, "Data in"=w12, "Guess parameters in"=w13) -> ("MLE_Baseline_Offset out"=w5:dbl, "All Parameter Constraints out"=w8:T10, "Data out"=w9:dbl[], "Guess parameters out"=w10:dbl[])  [unwired: 3 in]
  n24 = call "Get Fixed & Fitted Parameters.vi"("Error In"=w14, "All Parameter Constraints"=w8) -> ("Error Out"=w50:errorcluster, "All Parameter Constraints with Values"=w67:T24)  [unwired: 8 in]
  n25 = call "Get Fixed & Fitted Parameters v2.vi"("Error In"=w50, "Offset Resolution"=w53, "All Parameter Constraints with Values"=w67) -> ("Error Out"=w49:errorcluster, "Offset Array"=w43:dbl[], "Array of Fit Parameter Constraints with Values"=w66:T24[])  [unwired: 5 in, 1 out]
  n26 = for "For Loop on weights options" {
    tunnel: w79 -> [w152]
    tunnel: w78 -> [w151]
    tunnel: w9 -> [w150]
    tunnel: w47 -> [w148]
    tunnel: w28 -> [w147]
    tunnel: [w146] -> w18
    tunnel: [w145] -> w16
    tunnel: [w144] -> w70
    tunnel: w31 -> [w143]
    tunnel: w32 -> [w142]
    tunnel: w66 -> [w141]
    tunnel: w64 -> [w140] mode=indexing
    tunnel: [w149] -> w44
    tunnel: w7 -> [w139]
    tunnel: w62 -> [w138]
    tunnel: w61 -> [w137]
    shift-right: [w136] -> w37
    shift-left: T4[] [] -> [w135]
    shift-right: [w134] -> w39
    shift-left: T19[] [] -> [w133]
    tunnel: "VI Refnum" -> [w132]
    tunnel: w10 -> [w131]
    shift-right: [w130] -> _
    shift-left: cluster{"All Guess Parameters (w tau)":dbl[]}[] [] -> [w129]
    shift-right: [w128] -> w41
    shift-left: w42 -> [w127]
    shift-right: [w126] -> w55
    shift-left: w56 -> [w125]
    tunnel: [w124] -> w52
    tunnel: w49 -> [w123]
    tunnel: w43 -> [w122]
    shift-right: [w121] -> w38
    shift-left: w40 -> [w120]
    tunnel: [FALSE ("Abort Fit")] -> w34
    tunnel: [w117] -> w2
    n27 = call "Logical Processors Used.vi"() -> ("# Logical Processor Used"=w118:i32)  [unwired: 6 in]
    n28 = case shown="False" w125 {
      selector: w125 -> [w160 w448]
      tunnel: w152 -> [w187 _]
      tunnel: w151 -> [w186 _]
      tunnel: w150 -> [w185 _]
      tunnel: [w184 _] -> w149
      tunnel: w148 -> [w183 _]
      tunnel: w147 -> [w182 _]
      tunnel: [w181 _] -> w146
      tunnel: [w180 _] -> w145
      tunnel: [w179 _] -> w144
      tunnel: w143 -> [w178 _]
      tunnel: w142 -> [w177 _]
      tunnel: w141 -> [w176 _]
      tunnel: w140 -> [w175 _]
      tunnel: w139 -> [w174 _]
      tunnel: w138 -> [w173 _]
      tunnel: w137 -> [w172 _]
      tunnel: [w171 _] -> w136
      tunnel: w135 -> [w170 _]
      tunnel: [w169 _] -> w134
      tunnel: w133 -> [w168 _]
      tunnel: w132 -> [w167 _]
      tunnel: w131 -> [w166 _]
      tunnel: [w165 _] -> w130
      tunnel: w129 -> [w164 _]
      tunnel: [w163 _] -> w128
      tunnel: w127 -> [w162 _]
      tunnel: [w161 w448] -> w126
      tunnel: [w159 _] -> w124
      tunnel: w123 -> [w158 _]
      tunnel: w122 -> [w157 _]
      tunnel: [w156 _] -> w121
      tunnel: w120 -> [w155 _]
      tunnel: w118 -> [w154 _]
      tunnel: [w153 _] -> w117
      frame False {
        n29 = case shown="\"Weighted Fit\"" w175 {
          tunnel: w187 -> [w220 w333 _]
          tunnel: w186 -> [w219 w332 w412]
          tunnel: w185 -> [w218 w303 _]
          tunnel: [w189 w296 w444] -> w184
          tunnel: w183 -> [w217 w331 _]
          tunnel: w182 -> [w216 w330 _]
          tunnel: [_ _ w442] -> w181
          tunnel: [_ _ w439] -> w180
          tunnel: [_ _ w443] -> w179
          tunnel: w178 -> [_ _ w445]
          tunnel: w177 -> [w188 w294 w446]
          tunnel: w176 -> [w215 w329 _]
          tunnel: w174 -> [w214 w328 _]
          tunnel: w173 -> [w213 w327 _]
          tunnel: w172 -> [w212 w326 _]
          tunnel: [w211 w300 w417] -> w171
          tunnel: w170 -> [w198 w312 w447]
          tunnel: [w209 w324 w421] -> w169
          tunnel: w168 -> [w210 w325 w441]
          tunnel: w167 -> [w208 w323 _]
          tunnel: w166 -> [w207 w322 _]
          tunnel: [w205 w320 _] -> w165
          tunnel: w164 -> [w197 w311 w440]
          tunnel: [w200 w316 w424] -> w163
          tunnel: w162 -> [_ _ w424]
          tunnel: [w196 w310 w438] -> w161
          tunnel: w160 -> [_ _ w438]
          tunnel: [_ _ w425] -> w159
          tunnel: w158 -> [w204 w306 w414]
          tunnel: w157 -> [w202 w318 _]
          tunnel: [w195 w304 w419] -> w156
          tunnel: w155 -> [w194 w309 w423]
          tunnel: w154 -> [w193 w302 _]
          tunnel: [_ _ w413] -> w153
          frame "Unweighted Fit" {
            n30 = for "For Loop on offset parameters" {
              tunnel: w220 -> [w264]
              tunnel: [w252] -> w199
              tunnel: w219 -> [w250]
              tunnel: w218 -> [w251]
              tunnel: w217 -> [w263]
              tunnel: w216 -> [w262]
              tunnel: w215 -> [w261] mode=indexing
              tunnel: w204 -> [w260]
              tunnel: w214 -> [w246]
              tunnel: w213 -> [w249]
              tunnel: w212 -> [w248]
              tunnel: [w259] -> w203 mode=indexing if=w253
              tunnel: w208 -> [w247]
              tunnel: w207 -> [w258]
              tunnel: [w257] -> w200
              tunnel: [w256] -> w206 mode=indexing if=w253
              tunnel: [w255] -> w196
              tunnel: [w254] -> w201 mode=indexing if=w253
              tunnel: w202 -> [w254] mode=indexing
              workers-P: w193 -> [_]
              tunnel: [w244] -> w192 mode=indexing
              n31 = global read "Abort Fit Global.vi" "Abort Fit"() -> (w245:bool)
              n32 = case shown="False" w245 {
                selector: w245 -> [_ w293]
                tunnel: w264 -> [w291 _]
                tunnel: w263 -> [w289 _]
                tunnel: w262 -> [w288 _]
                tunnel: w261 -> [w285 _]
                tunnel: w260 -> [w284 w292]
                tunnel: [w282 _] -> w259
                tunnel: w258 -> [w280 _]
                tunnel: [w279 _] -> w257
                tunnel: [w277 _] -> w256
                tunnel: [w276 w293] -> w255
                tunnel: [w275 _] -> w252
                tunnel: w251 -> [w270 _]
                tunnel: w250 -> [w271 _]
                tunnel: w249 -> [w269 _]
                tunnel: w248 -> [w268 _]
                tunnel: w247 -> [w266 _]
                tunnel: w246 -> [w267 _]
                tunnel: [w265 w292] -> w244
                frame False {
                  # "sigma = sqrt(abs(tau))"
                  # "not aborted"
                  n33 = Unbundle By Name(w285) -> ("Fit Model"=w287:T12, "Fixed Parameter Names"=w279:T11[], "Fixed Parameter Values"=w272:dbl[], "Fitted Parameter Names"=w286:T11[], "Fitted parameter bounds"=w273:T21)
                  n34 = node(w288) -> (w290:dbl)
                  n35 = Bundle By Name(cluster=T19 {"IRF"={"X Array"=[], "Y Array"=[]}, "Laser Period"=0.0, "SYNC Period"=0.0, "Fixed Parameter Names"=[], "Fixed Parameter Values"=[], "Fitted Parameter Names"=[], "Fit Model"=enum."1-Exponential"}, "Laser Period"=w291, "SYNC Period"=w290, "IRF"=w289, "Fit Model"=w287, "Fixed Parameter Names"=w279, "Fixed Parameter Values"=w272, "Fitted Parameter Names"=w286) -> (w275:T19)
                  n36 = call "Replace Fixed Parameters.vi"("Fit Model"=w287, "Error In"=w284, "Fixed Parameter Values (w sigma)"=w272, "Fixed Parameter Names"=w279, "All Guess Parameters in (w tau)"=w280) -> ("Error Out"=w283:errorcluster, "Guess Fitted Parameters (w sigma)"=w274:dbl[], "All Guess Parameters (w tau)"=w278:dbl[])  [unwired: 2 in, 2 out]
                  n37 = Bundle("All Guess Parameters (w tau)"=w278) -> (w277:cluster{"All Guess Parameters (w tau)":dbl[]})  [unwired: 1 in]
                  n38 = call "Constrained Non-Linear Fit (Best of All).vi"("Y Array"=w270, "f(x,a)"=w266, "Data"=w275, "Fitting Method"=w267, "X Array"=w271, "Guess Fitted Parameters"=w274, "error in (no error)"=w283, "Termination Criteria"=w269, "Fitted parameter bounds"=w273, "Fitting Algorithm"=w268) -> ("Fit Output"=w282:T4, "Fit Aborted?"=w276:bool, "Error Out"=w265:errorcluster)  [unwired: 2 in, 1 out]
                }
                frame True {
                  # "Fit aborted"
                }
              }
              n39 = Not(x=w255) -> (.not. x?=w253:bool)
            }
            n40 = Merge Errors(w192) -> (w191:errorcluster)
            n41 = call "Clear Error.vi"("Error In"=w191) -> ("no Error Out"=w190:errorcluster)  [unwired: 8 in]
            n42 = case shown="False" w196 {
              tunnel: [w238 w242] -> w211
              tunnel: w210 -> [w237 w243]
              tunnel: [w236 w243] -> w209
              tunnel: w206 -> [w235 _]
              tunnel: [w234 w241] -> w205
              tunnel: w203 -> [w233 _]
              tunnel: w201 -> [w232 _]
              tunnel: w199 -> [w224 _]
              tunnel: w198 -> [w230 w242]
              tunnel: w197 -> [w229 w241]
              tunnel: [w227 w240] -> w195
              tunnel: w194 -> [w226 w240]
              tunnel: w190 -> [w223 w239]
              tunnel: [w222 w239] -> w189
              tunnel: w188 -> [w221 _]
              frame False {
                # "not aborted"
                n43 = call "Compute N-Exp Fit Optimal Offset.vi"("Fit Control Data in"=w224, "Error In"=w223, "Offset Array"=w232, "Decay Normalization Factor"=w221, "Fit Output in"=w233) -> ("Error Out"=w222:errorcluster, "C_00"=w228:dbl, "Fit Output out"=w231:T4, "Fit Control Data out"=w225:T19)  [unwired: 3 in]
                n44 = Build Array (concatenate)(w237, w225) -> (w236:T19[])
                n45 = Build Array (concatenate)(w229, w235) -> (w234:cluster{"All Guess Parameters (w tau)":dbl[]}[])
                n46 = Build Array (concatenate)(w230, w231) -> (w238:T4[])
                n47 = Build Array (concatenate)(w226, w228) -> (w227:dbl[])
              }
              frame True {
                # "Fit aborted"
              }
            }
          }
          frame "Weighted Fit" {
            # "Restores scaled\nvalues for fitting"
            # "Restores original\nvalues for weights\nevaluation"
            n48 = Compound Arithmetic op=MULTIPLY(w294, w303) -> (w295:dbl[])
            n49 = call "Compute Weight Array v2.vi"("Error In"=w306, "Weighted Fit"=TRUE, "Data Array"=w295) -> ("Error Out"=w307:errorcluster, "Weight Array"=w305:dbl[])  [unwired: 7 in]
            n50 = Compound Arithmetic op=MULTIPLY(invert w294, w305) -> (w301:dbl[])
            n51 = for "For Loop on offset parameters" {
              tunnel: w333 -> [w378]
              tunnel: [w366] -> w315
              tunnel: w332 -> [w364]
              tunnel: w303 -> [w365]
              tunnel: w331 -> [w377]
              tunnel: w330 -> [w376]
              tunnel: w329 -> [w375] mode=indexing
              tunnel: w307 -> [w374]
              tunnel: w328 -> [w360]
              tunnel: w327 -> [w363]
              tunnel: w326 -> [w362]
              tunnel: [w373] -> w319 mode=indexing if=w367
              tunnel: w323 -> [w361]
              tunnel: w322 -> [w372]
              tunnel: [w371] -> w316
              tunnel: [w370] -> w321 mode=indexing if=w367
              tunnel: [w369] -> w310
              tunnel: [w368] -> w317 mode=indexing if=w367
              tunnel: w318 -> [w368] mode=indexing
              tunnel: [w361] -> w314
              tunnel: [w360] -> w313
              tunnel: w301 -> [w358]
              workers-P: w302 -> [_]
              tunnel: [w357] -> w299 mode=indexing
              n52 = global read "Abort Fit Global.vi" "Abort Fit"() -> (w359:bool)
              n53 = case shown="False" w359 {
                selector: w359 -> [_ w410]
                tunnel: w378 -> [w406 _]
                tunnel: w377 -> [w404 _]
                tunnel: w376 -> [w403 _]
                tunnel: w375 -> [w400 _]
                tunnel: w374 -> [w399 w407]
                tunnel: [w397 _] -> w373
                tunnel: w372 -> [w395 _]
                tunnel: [w393 _] -> w371
                tunnel: [w391 _] -> w370
                tunnel: [w390 w410] -> w369
                tunnel: [w389 _] -> w366
                tunnel: w365 -> [w382 _]
                tunnel: w364 -> [w383 _]
                tunnel: w363 -> [w381 _]
                tunnel: w362 -> [w380 _]
                tunnel: w361 -> [w385 w409]
                tunnel: w360 -> [w384 w408]
                tunnel: w358 -> [w386 _]
                tunnel: [w385 w409] -> _
                tunnel: [w384 w408] -> _
                tunnel: [w379 w407] -> w357
                frame False {
                  # "sigma = sqrt(abs(tau))"
                  # "not aborted"
                  n54 = Unbundle By Name(w400) -> ("Fit Model"=w402:T12, "Fixed Parameter Names"=w393:T11[], "Fixed Parameter Values"=w394:dbl[], "Fitted Parameter Names"=w401:T11[], "Fitted parameter bounds"=w387:T21)
                  n55 = node(w403) -> (w405:dbl)
                  n56 = Bundle By Name(cluster=T19 {"IRF"={"X Array"=[], "Y Array"=[]}, "Laser Period"=0.0, "SYNC Period"=0.0, "Fixed Parameter Names"=[], "Fixed Parameter Values"=[], "Fitted Parameter Names"=[], "Fit Model"=enum."1-Exponential"}, "Laser Period"=w406, "SYNC Period"=w405, "IRF"=w404, "Fit Model"=w402, "Fixed Parameter Names"=w393, "Fixed Parameter Values"=w394, "Fitted Parameter Names"=w401) -> (w389:T19)
                  n57 = call "Replace Fixed Parameters.vi"("Fit Model"=w402, "Error In"=w399, "Fixed Parameter Values (w sigma)"=w394, "Fixed Parameter Names"=w393, "All Guess Parameters in (w tau)"=w395) -> ("Error Out"=w398:errorcluster, "Guess Fitted Parameters (w sigma)"=w388:dbl[], "All Guess Parameters (w tau)"=w392:dbl[])  [unwired: 2 in, 2 out]
                  n58 = Bundle("All Guess Parameters (w tau)"=w392) -> (w391:cluster{"All Guess Parameters (w tau)":dbl[]})  [unwired: 1 in]
                  n59 = call "Constrained Non-Linear Fit (Best of All).vi"("Y Array"=w382, "f(x,a)"=w385, "Data"=w389, "Fitting Method"=w384, "X Array"=w383, "Weights"=w386, "Guess Fitted Parameters"=w388, "error in (no error)"=w398, "Termination Criteria"=w381, "Fitted parameter bounds"=w387, "Fitting Algorithm"=w380) -> ("Fit Output"=w397:T4, "Fit Aborted?"=w390:bool, "Error Out"=w379:errorcluster)  [unwired: 1 in, 1 out]
                }
                frame True {
                  # "fit aborted"
                }
              }
              n60 = Not(x=w369) -> (.not. x?=w367:bool)
            }
            n61 = Merge Errors(w299) -> (w298:errorcluster)
            n62 = call "Clear Error.vi"("Error In"=w298) -> ("no Error Out"=w297:errorcluster)  [unwired: 8 in]
            n63 = case shown="False" w310 {
              tunnel: [w351 w355] -> w300
              tunnel: w325 -> [w350 w356]
              tunnel: [w349 w356] -> w324
              tunnel: w321 -> [w348 _]
              tunnel: [w347 w354] -> w320
              tunnel: w319 -> [w346 _]
              tunnel: w317 -> [w345 _]
              tunnel: w315 -> [w344 _]
              tunnel: w314 -> [_ _]
              tunnel: w313 -> [_ _]
              tunnel: w312 -> [w342 w355]
              tunnel: w311 -> [w341 w354]
              tunnel: w309 -> [w339 w353]
              tunnel: [w338 w353] -> w304
              tunnel: w297 -> [w336 w352]
              tunnel: [w335 w352] -> w296
              tunnel: w294 -> [w334 _]
              frame False {
                # "not aborted"
                n64 = call "Compute N-Exp Fit Optimal Offset.vi"("Fit Control Data in"=w344, "Error In"=w336, "Offset Array"=w345, "Decay Normalization Factor"=w334, "Fit Output in"=w346) -> ("Error Out"=w335:errorcluster, "C_00"=w340:dbl, "Fit Output out"=w343:T4, "Fit Control Data out"=w337:T19)  [unwired: 3 in]
                n65 = Build Array (concatenate)(w350, w337) -> (w349:T19[])
                n66 = Build Array (concatenate)(w342, w343) -> (w351:T4[])
                n67 = Build Array (concatenate)(w341, w348) -> (w347:cluster{"All Guess Parameters (w tau)":dbl[]}[])
                n68 = Build Array (concatenate)(w339, w340) -> (w338:dbl[])
              }
              frame True {
                # "fit aborted"
              }
            }
          }
          frame "Best Fit" {
            # "---normalized amplitudes, parameters with sigma -------------------------------------->"
            # "---unscaled amplitudes -------------------------------------->"
            n69 = Array Size(array=w412) -> (size(s)=w411:i32)
            n70 = call "Get Best Fit Output v2.vi"("error in"=w414, "Array of Fit Outputs"=w447) -> ("Error Out"=w427:errorcluster, "max index"=w422:i32, "Best Fit Output"=w437:T4)  [unwired: 7 in]
            n71 = Index Array(array=w423, index=w422) -> (element=w420:dbl)
            n72 = Index Array(array=w441, index=w422) -> (element=w416:T19)
            n73 = Index Array(array=w440, index=w422) -> (element=w426:cluster{"All Guess Parameters (w tau)":dbl[]})
            n74 = call "1D Fit Unscale Fit Outputs v2.vi"("# Points"=w411, "Fit Control Data in"=w416, "Error In"=w427, "IRF Normalization Factor"=w445, "Decay Normalization Factor"=w446, "Fit Output in  (w sigma)"=w437) -> ("Error Out"=w444:errorcluster, "All unscaled parameters (w tau)"=w442:dbl[], "Fitted unscaled parameters (w tau)"=w413:dbl[], "Unscaled Fit Output out (w sigma)"=w418:T4, "Fit Control Data out"=w415:T19)  [unwired: 1 in]
            n75 = Unbundle(w426) -> ("All Guess Parameters (w tau)"=w439:dbl[])
            n76 = Unbundle By Name(w418) -> ("Fitting Algorithm"=w430:T8, "Fitting Method"=w434:T5, "R^2"=w433:dbl, "RMSE"=w432:dbl, "Chi 2"=w431:dbl, "DOF"=w429:i32, "Weighted Fit"=w425:bool)
            n77 = Divide(x=w431, y=w429) -> (x/y=w428:dbl)
            n78 = Bundle By Name(cluster=T25 {"Chi2/DOF"=0.0, "R2"=0.0, "RMSE"=0.0, "Fitting Method"=enum."Least Square", "Fitting Algorithm"=enum."Levenberg-Marquardt"} ("Fit Results (Stats)"), "Fitting Algorithm"=w430, "Fitting Method"=w434, "R2"=w433, "RMSE"=w432, "Chi2/DOF"=w428) -> (w435:T25)
            n79 = Build Array(w435) -> (w443:T25[])
            n80 = Build Array(w420) -> (w419:dbl[])
            n81 = Build Array(w415) -> (w421:T19[])
            n82 = Build Array(w418) -> (w417:T4[])
          }
        }
      }
      frame True {
      }
    }
  }
  n83 = Index Array(array=w38) -> (element=w36:dbl)  [unwired: 1 in]
  n84 = Index Array(array=w39) -> (element=w22:T19)  [unwired: 1 in]
  n85 = Index Array(array=w37) -> (element=w21:T4)  [unwired: 1 in]
  n86 = global write "Abort Fit Global.vi" "Abort Fit"(w34) -> ()
  n87 = Square Root(x=w36) -> (sqrt(x)=w35:dbl)
  n88 = call "Downshift MLE Baseline.vi"("Fit Control Data in"=w22, "NL Fit Method"=w7, "IRF"="IRF", "rescaled, w sigma"=w21, "Fitted unscaled parameters w tau"=w2, "all unscaled parameters w tau"=w18, "All Guess Parameters w tau"=w16, "MLE_Baseline_Shift"=w5) -> ("Fit Control Data out"=w20:T19, "Fit Output"=w19:T4, "Fitted unscaled parameters w tau"=w1:dbl[], "All unscaled Parameters (w tau)"=w17:dbl[], "All Guess Parameters (w tau)"=→"Guess Parameters":dbl[])  [unwired: 3 in]
  n89 = case shown="False" w55 {
    tunnel: [w492 _] -> w86
    tunnel: [w491 _] -> w85
    tunnel: [w463 w525] -> w84
    tunnel: [w457 w520] -> w83
    tunnel: [w490 _] -> w82
    tunnel: "VI Refnum" -> [w487 _]
    tunnel: w19 -> [w449 w524]
    tunnel: [w449 w523] -> w80
    tunnel: w44 -> [w482 _]
    tunnel: w70 -> [w474 _]
    tunnel: w17 -> [w452 _]
    tunnel: w41 -> [w453 _]
    tunnel: w58 -> [w468 _]
    tunnel: w59 -> [w467 _]
    tunnel: "IRF" -> [w462 _]
    tunnel: "Decay" -> [w461 _]
    tunnel: w20 -> [w450 _]
    tunnel: w45 -> [w459 w521]
    tunnel: w52 -> [w458 _]
    tunnel: w35 -> [w455 _]
    tunnel: [w452 w520] -> w33
    tunnel: w1 -> [w451 _]
    frame False {
      w479 = TRUE ("Get(F)/Set")
      # "reset decay to its unscaled values"
      # "reset IRF to its unscaled values"
      # "Fixed parameters have an uncertainty of 0"
      n90 = Unbundle By Name(w461) -> ("Data Array"=w465:dbl[], "t Array"=w456:dbl[])
      n91 = Array Max & Min(array=w465) -> (max value=w477:dbl, min value=w476:dbl)  [unwired: 2 out]
      n92 = call "AlliGator Update Decay Fit Results (Stats).vi"("error in (no error)"=w482, "Fit Results"=w474) -> ("error out"=w481:errorcluster)  [unwired: 9 in]
      n93 = Unbundle By Name(w449) -> ("best nonlinear fit"=w486:dbl[])  [unwired: 1 out]
      n94 = call "Model Parameter List.vi"("Fit Model"=w459) -> ("Model Parameter List"=w460:T11[])
      n95 = Subtract(x=w477, y=w476) -> (x-y=w475:dbl)
      n96 = Bundle By Name(cluster=w450, "IRF"=w462) -> ()  [unwired: 1 out]
      n97 = call "Alligator Variables Storage.vi"("Get(F)/Set"=w479, "AlliGator Variable"=AlliGator_Variables_List."Last Decay Max - Min" ("Alligator Variable"), "Error In"=w481, "Data in"=w475) -> ("Error Out"=w480:errorcluster)  [unwired: 5 in, 2 out]
      n98 = call "Compute Weight Array v2.vi"("Weighted Fit"=w458, "Data Array"=w465) -> ("Weight Array"=w466:dbl[])  [unwired: 8 in, 1 out]
      n99 = call "Alligator Variables Storage.vi"("Get(F)/Set"=w479, "AlliGator Variable"=AlliGator_Variables_List."Best Fit Parameters" ("Alligator Variable"), "Error In"=w480, "Data in"=w452) -> ("Error Out"=w484:errorcluster)  [unwired: 5 in, 2 out]
      n100 = Subtract(x=w465, y=w486) -> (x-y=w489:dbl[])
      n101 = case shown="\"Reduced\"" w468 {
        tunnel: w489 -> [w511 w514 w519]
        tunnel: [w511 w512 w517] -> w488
        tunnel: w486 -> [_ w513 w518]
        frame "Standard", Default {
        }
        frame "Normalized" {
          n102 = Divide(x=w514, y=w513) -> (x/y=w512:dbl[])
        }
        frame "Reduced" {
          n103 = Absolute Value(x=w518) -> (abs(x)=w516:dbl[])
          n104 = Square Root(x=w516) -> (sqrt(x)=w515:dbl[])
          n105 = Divide(x=w519, y=w515) -> (x/y=w517:dbl[])
        }
      }
      n106 = call "Alligator Variables Storage.vi"("Get(F)/Set"=w479, "AlliGator Variable"=AlliGator_Variables_List."Best Fit Parameter Names" ("Alligator Variable"), "Error In"=w484, "Data in"=w460) -> ("Error Out"=w473:errorcluster)  [unwired: 5 in, 2 out]
      n107 = Compound Arithmetic op=MULTIPLY(w453, 0.0 ("value")) -> (w470:dbl[])
      n108 = case shown="True" w467 {
        tunnel: [w496 w499] -> w471
        tunnel: [w493 w500] -> w472
        tunnel: w456 -> [_ w509]
        tunnel: w487 -> [_ w508]
        tunnel: w466 -> [_ w507]
        tunnel: w450 -> [_ w506]
        tunnel: w473 -> [w496 w499]
        tunnel: w451 -> [w494 w498]
        tunnel: w465 -> [_ w497]
        frame False {
          n109 = Compound Arithmetic op=MULTIPLY(0.0, w494) -> (w493:dbl[])
        }
        frame True {
          n110 = Array Size(array=w498) -> (size(s)=w505:i32)
          n111 = call "My Nonlinear Curve Fit Intervals.vi"("Y"=w497, "confidence level"=0.68, "f(x,a)"=w508, "data"=w506, "X"=w509, "Weight"=w507, "best fit parameters"=w498, "error in (no error)"=w499) -> ("delta best fit parameters"=w501:dbl[], "error out"=w502:errorcluster)  [unwired: 6 in]
          n112 = Initialize Array(nan ("element"), w505) -> (w503:dbl[])
          n113 = Select(t=w503, s=w502, f=w501) -> (s? t:f=w500:dbl[])
        }
      }
      n114 = Bundle("t Array"=w456, "best nonlinear fit"=w486) -> (w491:T27)  [unwired: 1 in]
      n115 = Bundle("t Array"=w456, w488) -> (w490:cluster{"t Array":dbl[], dbl[]})  [unwired: 1 in]
      n116 = call "1D Fit Insert Fixed Parameters.vi"("Fit Model"=w459, "Error In"=w471, "Fixed Parameter Names"=w453, "Fixed Parameter Values"=w470, "Fitted Parameters"=w472) -> ("Error Out"=w463:errorcluster, "All Parameters"=w464:dbl[])  [unwired: 5 in]
      n117 = Build Array(w462, w461, w491, w490) -> (w492:T18)
      n118 = Replace Array Subset(array=w464, new element=w455, index=0) -> (w457:dbl[])
    }
    frame True {
      w522 = nan ("element")
      # "Fit Aborted by user"
      n119 = case shown="\"1-Exponential\", Default" w521 {
        tunnel: [4 ("dimension size") 6 ("dimension size")] -> w526
        frame "1-Exponential", Default {
        }
        frame "2-Exponentials" {
        }
      }
      n120 = xnode "Error Ring"() -> ("error out"=w525:errorcluster)
      n121 = Initialize Array(w522, w526) -> (w520:dbl[])
      n122 = Bundle By Name(cluster=w524, "best nonlinear fit"=w520, "best fit parameters"=w520, "R^2"=w522, "RMSE"=w522) -> (w523:T4)
    }
  }
  "Fitted Decay" <- w85
  "XY Graph" <- w86
  "Delta Best Fit Parameters (w tau)" <- w83
  "Residuals" <- w82
  "Fit Output" <- w80
  "All unscaled Fit Parameters (w tau)" <- w33
  n123 = call "High Resolution Timing.vi"("relative seconds (NaN)"=w63, "Error In"=w84) -> ("elapsed (relative) seconds"=→"CPU (s)":dbl, "Error Out"=→"error out":errorcluster)  [unwired: 15 in, 1 out]
